vi "Angle to PWM Time.vi"(11 "Angle (degrees)":dbl) -> (3 "PWM value":dbl)   [LabVIEW 2015]
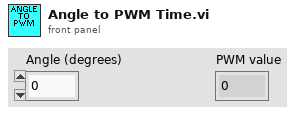
[diagram p1: front panel]
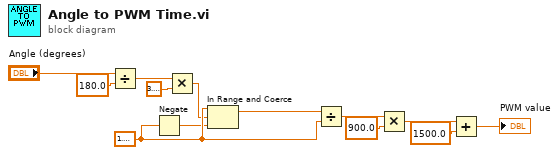
[diagram p0: block diagram]
diagram:
  w7 = 1.5707963267948966
  n1 = Divide(x="Angle (degrees)", y=180.0) -> (x/y=w4:dbl)
  n2 = Negate(x=w7) -> (-x=w5:dbl)
  n3 = Multiply(x=w4, y=3.141592653589793) -> (x*y=w3:dbl)
  n4 = In Range and Coerce(upper limit=w7, x=w3, lower limit=w5) -> (coerced(x)=w6:dbl)  [unwired: 1 out]
  n5 = Divide(x=w6, y=w7) -> (x/y=w8:dbl)
  n6 = Multiply(x=w8, y=900.0) -> (x*y=w10:dbl)
  n7 = Add(x=w10, y=1500.0) -> (x+y=→"PWM value":dbl)
